vi "UIOutputToString.vi"(8 "ErrorIn":errorcluster, 11 "UIOutput":T1) -> (0 "ErrorOut":errorcluster, 3 "String":string)   [LabVIEW 2019]
uses:
  MobileAnalyzer/mainVIs/UIVIs/UIOutput.ctl
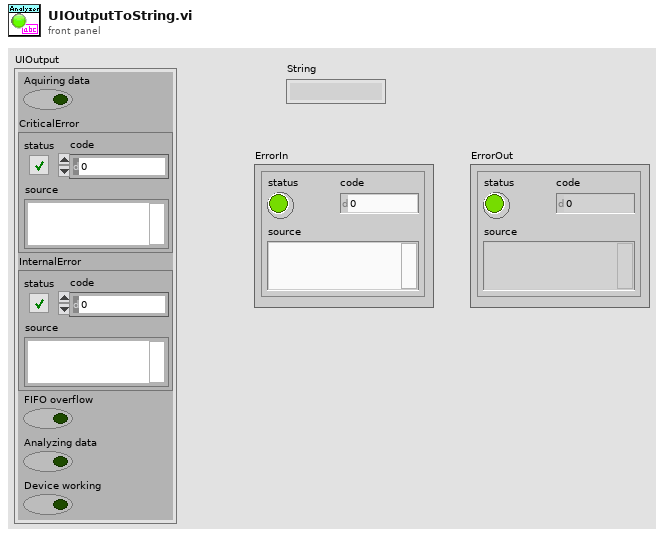
[diagram p1: front panel]
types:
  T1 = typedef "UIOutput.ctl" = cluster{"Aquiring data":bool, "CriticalError":errorcluster, "InternalError":errorcluster, "FIFO overflow":bool, "Analyzing data":bool, "Device working":bool}
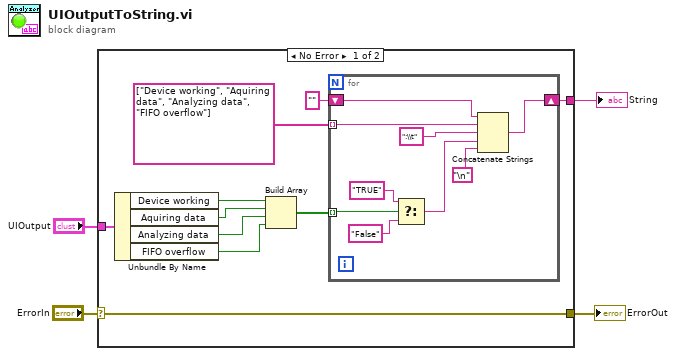
[diagram p0: block diagram]
diagram:
  n1 = case shown="No Error" "ErrorIn" {
    selector: "ErrorIn" -> [w5 w24]
    tunnel: "UIOutput" -> [w14 _]
    tunnel: [w6 _] -> w3
    tunnel: [w5 w24] -> w1
    frame No Error {
      n2 = Unbundle By Name(w14) -> ("Device working"=w13:bool, "Aquiring data"=w10:bool, "Analyzing data"=w11:bool, "FIFO overflow"=w12:bool)
      n3 = Build Array(w13, w10, w11, w12) -> (w9:bool[])
      n4 = for {
        tunnel: w9 -> [w23] mode=indexing
        tunnel: string[] ["Device working", "Aquiring data", "Analyzing data", "FIFO overflow"] -> [w20] mode=indexing
        shift-right: [w16] -> w6
        shift-left: "" -> [w15]
        n5 = Select(t="TRUE" ("String"), s=w23, f="False" ("String")) -> (s? t:f=w18:string)
        n6 = Concatenate Strings(w15, w20, ":\\t" ("string"), w18, "\n") -> (w16:string)
      }
    }
    frame Error {
    }
  }
  "String" <- w3
  "ErrorOut" <- w1
